vi "Read Paths.vi"() -> (3 "Paths":map{string, dbl[][]}(c390))   [LabVIEW 2019]
uses:
  Drive Published Globals.vi
  <vilib>/Utility/file.llb/Read Delimited Spreadsheet (DBL).vi
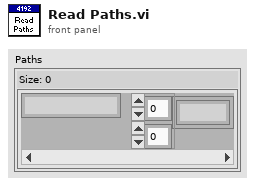
[diagram p1: front panel]
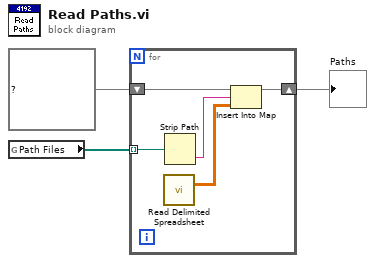
[diagram p0: block diagram]
diagram:
  n1 = global read "Drive Published Globals.vi" "Path Files"() -> (w2:path[])
  n2 = for {
    shift-right: [w7] -> w1
    shift-left: map{string, dbl[][]} {} ("Map") -> [w8]
    tunnel: w2 -> [w5] mode=indexing
    n3 = call-poly <vilib>:"Read Delimited Spreadsheet.vi"() -> ("all rows"=w6:dbl[][])  [unwired: 10 in, 5 out]
    n4 = Strip Path(path=w5) -> (name=w4:string)  [unwired: 1 out]
    n5 = Insert Into Map(map in=w8, key=w4, value=w6) -> (map out=w7:map{string, dbl[][]})  [unwired: 2 out]
  }
  "Paths" <- w1
